vi "GenerateDictionaryFromVIs.vi"(7 "VIs in":refnum<vi>[](array[refnum]), 8 "error in (no error)":errorcluster, 10 "Additional Languages [English]":string[](array[string])=["English"], 11 "Current VI Language (English)":string="English") -> (0 "error out":errorcluster, 3 "Localization":T1)   [LabVIEW 2019]
uses:
  Dictionary--Cluster.ctl
  Font -- Cluster.ctl
  Phrase Dictionary Entry -- Cluster.ctl
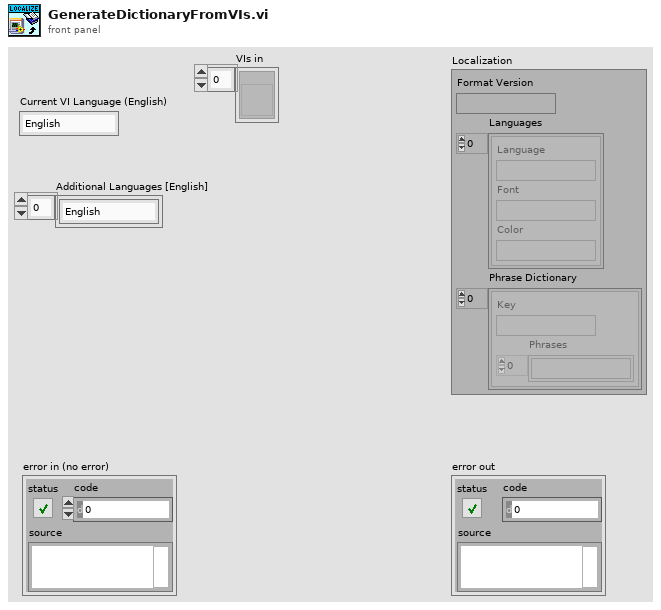
[diagram p1: front panel]
types:
  T1 = typedef "Dictionary--Cluster.ctl" = cluster{"Format Version":string, "Languages":T2[], "Phrase Dictionary":T3[]}
  T2 = typedef "Font -- Cluster.ctl" = cluster{"Language":string, "Font":string, "Color":string}
  T3 = typedef "Phrase Dictionary Entry -- Cluster.ctl" = cluster{"Key":string, "Phrases":string[]}
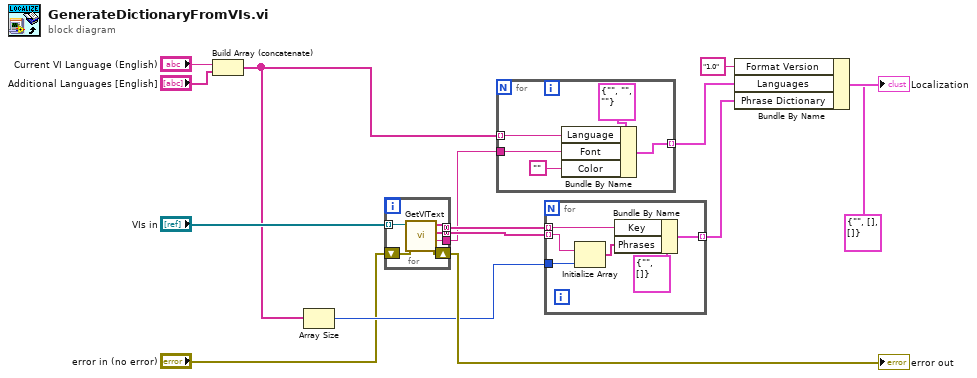
[diagram p0: block diagram]
diagram:
  n1 = Build Array (concatenate)("Current VI Language (English)", "Additional Languages [English]") -> (w4:string[])
  n2 = Array Size(array=w4) -> (size(s)=w13:i32)
  n3 = for {
    tunnel: "VIs in" -> [w21] mode=indexing
    tunnel: [w20] -> w10 mode=concatenating
    tunnel: [w19] -> w9 mode=concatenating
    shift-right: [w18] -> w15
    shift-left: "error in (no error)" -> [w17]
    tunnel: [w16] -> w3
    n4 = call "GetVIText.vi"("error in (no error)"=w17, "VI"=w21) -> ("error out"=w18:errorcluster, "Font Name"=w16:string, "Control Text"=w20:string[], "Control Keys"=w19:string[])  [unwired: 5 in, 1 out]
  }
  "error out" <- w15
  n5 = for {
    tunnel: w4 -> [w25] mode=indexing
    tunnel: w3 -> [w24]
    tunnel: [w23] -> w2 mode=indexing
    n6 = Bundle By Name(cluster=T2 {"Language"="", "Font"="", "Color"=""} ("Font"), "Language"=w25, "Font"=w24, "Color"="") -> (w23:T2)
  }
  n7 = for {
    tunnel: w9 -> [w31] mode=indexing
    tunnel: w10 -> [w29] mode=indexing
    tunnel: w13 -> [w30]
    tunnel: [w27] -> w8 mode=indexing
    n8 = Initialize Array(w29, w30) -> (w28:string[])
    n9 = Bundle By Name(cluster=T3 {"Key"="", "Phrases"=[]} ("Phrase Dictionary"), "Key"=w31, "Phrases"=w28) -> (w27:T3)
  }
  n10 = Bundle By Name(cluster=T1 {"Format Version"="", "Languages"=[], "Phrase Dictionary"=[]} ("Localization"), "Format Version"="1.0", "Languages"=w2, "Phrase Dictionary"=w8) -> (→"Localization":T1)
